vi "create libtls server.vi"(8 "error in":errorcluster) -> (0 "error out":errorcluster, 3 "server out":u64)   [LabVIEW 2016, in "lv tls dll.lvlib"]
uses:
  lv tls dll.lvlib
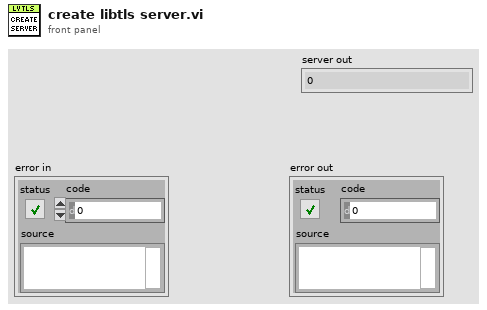
[diagram p1: front panel]
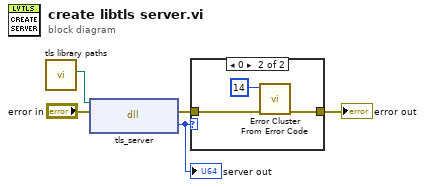
[diagram p0: block diagram]
diagram:
  n1 = call "tls library paths.vi"() -> ("libtls"=w5:path)  [unwired: 8 in, 3 out]
  n2 = dll-call lib="C:/Users/IEUser/Desktop/tlssimple/libtls-15.dll" fn="tls_server"(path in=w5, error in="error in") -> (error out=w3:errorcluster, "server"=w1:u64)  [unwired: 1 in, 1 out]
  "server out" <- w1
  n3 = case shown="0" w1 {
    tunnel: w3 -> [w6 w9]
    tunnel: [w6 w8] -> w2
    frame Default {
    }
    frame 0 {
      n4 = call <vilib>:"Error Cluster From Error Code.vi"("error in (no error)"=w9, "error code (0)"=14) -> ("error out"=w8:errorcluster)  [unwired: 7 in]
    }
  }
  "error out" <- w2
